vi "RUN_ALL_TESTS.vi"() -> (0 "All_Test_passed":bool)   [LabVIEW 2015]
panel:
  out "Test_OK":bool[](array[boolean])=[TRUE, FALSE]
  # "Test basic methods with some testing plant"
  # "Open"
  # "Close"
  # "Start"
  # "Stop"
  # "Get"
  # "Set"
  # "Multiple formats set-get"
  # "Functional Test"
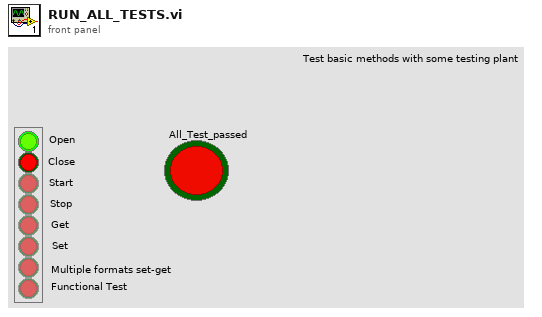
[diagram p1: front panel]
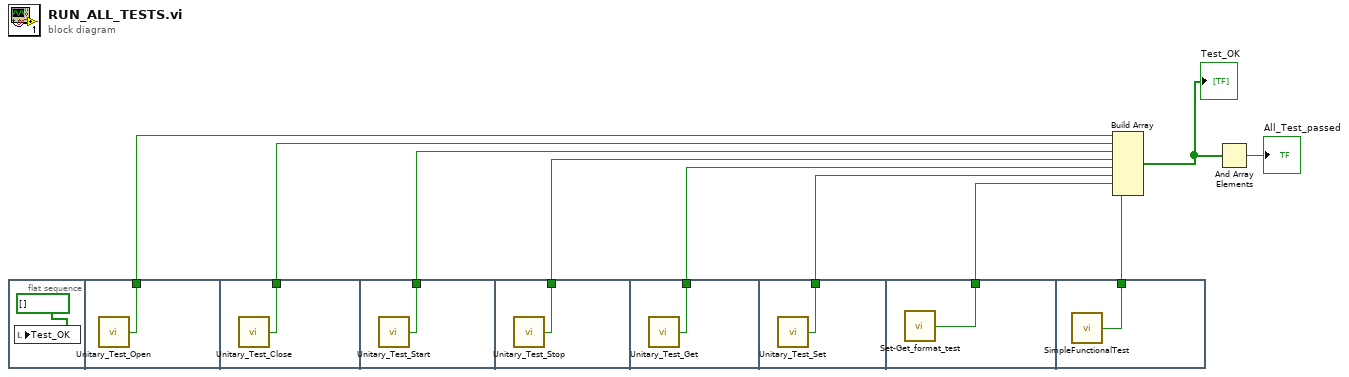
[diagram p0: block diagram]
diagram:
  n1 = flat-sequence {
    tunnel: [w12] -> w8
    tunnel: [w13] -> w7
    tunnel: [w14] -> w6
    tunnel: [w15] -> w5
    tunnel: [w16] -> w4
    tunnel: [w17] -> w3
    tunnel: [w18] -> w1
    tunnel: [w19] -> w2
    frame #0 {
      n2 = local write "Test_OK"(bool[] [] ("appended array")) -> ()
    }
    frame #1 {
      n3 = call "Unitary_Test_Open.vi"() -> ("Test_passed"=w12:bool)
    }
    frame #2 {
      n4 = call "Unitary_Test_Close.vi"() -> ("Test_passed"=w13:bool)
    }
    frame #3 {
      n5 = call "Unitary_Test_Start.vi"() -> ("Test_passed"=w14:bool)
    }
    frame #4 {
      n6 = call "Unitary_Test_Stop.vi"() -> ("Test_passed"=w15:bool)
    }
    frame #5 {
      n7 = call "Unitary_Test_Get.vi"() -> ("Test_passed"=w16:bool)
    }
    frame #6 {
      n8 = call "Unitary_Test_Set.vi"() -> ("Test_passed"=w17:bool)
    }
    frame #7 {
      n9 = call "Set-Get_format_test.vi"() -> ("Test_passed"=w18:bool)
    }
    frame #8 {
      n10 = call "SimpleFunctionalTest.vi"() -> ("test OK"=w19:bool)
    }
  }
  n11 = Build Array(w8, w7, w6, w5, w4, w3, w1, w2) -> (w9:bool[])
  "Test_OK" <- w9
  n12 = And Array Elements(Boolean array=w9) -> (logical AND=→"All_Test_passed":bool)
